vi "Array.vi"() -> ()   [LabVIEW 2018]
panel:
  out "배열연결이지만 입력연결 안한것 (차원이 늘어남)":dbl[][](array[numeric])
  out "상수와 배열의 연결":dbl[](array[numeric])
  out "입력연결 한것 (배열 뒤로 연결)":dbl[](array[numeric])
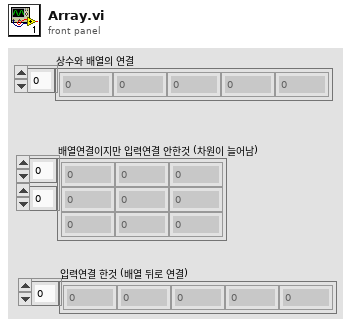
[diagram p1: front panel]
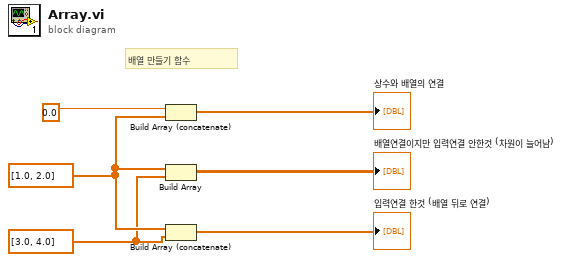
[diagram p0: block diagram]
diagram:
  w4 = dbl[] [3.0, 4.0]
  w5 = dbl[] [1.0, 2.0]
  # "배열 만들기 함수"
  n1 = Build Array (concatenate)(0.0, w5) -> (→"상수와 배열의 연결":dbl[])
  n2 = Build Array(w5, w4) -> (→"배열연결이지만 입력연결 안한것 (차원이 늘어남)":dbl[][])
  n3 = Build Array (concatenate)(w5, w4) -> (→"입력연결 한것 (배열 뒤로 연결)":dbl[])
